vi "Query Limit Test Status.vi"(8 "error in (no error)":errorcluster, 9 "Limit Number (1: Limit 1)":i32(ring)=1 items=["Limit 1"=1, "Limit 2"=2], 10 "Function (0: Voltage DC)":i32(ring) items=["Voltage DC", "Voltage AC", "Current DC", "Current AC", "Resistance", "4-wire Resistance", "Diode", "Capacitance", "Temperature", "Continuity", "Frequency", "Period", "Voltage Ratio", "Digitize Voltage", "Digitize Current"], 11 "VISA resource name":refnum<visa-resource-name>) -> (0 "error out":errorcluster, 1 "Pass":bool, 2 "Fail Reason":string, 3 "VISA resource name out":refnum<visa-resource-name>)   [LabVIEW 2023, in "Keithley DMM6500 DAQ6500 Series.lvlib"]
doc: "Queries if the test result for limit Y should be cleared automatically or not."
uses:
  <instrlib>/Keithley DMM6500 DAQ6500 Series/Keithley DMM6500 DAQ6500 Series.lvlib
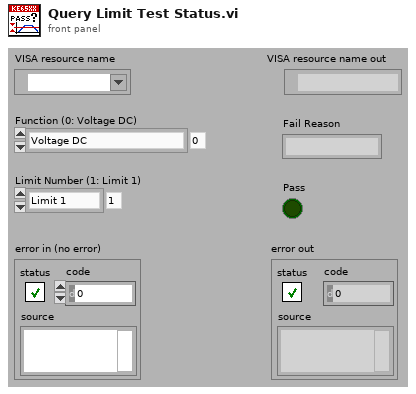
[diagram p1: front panel]
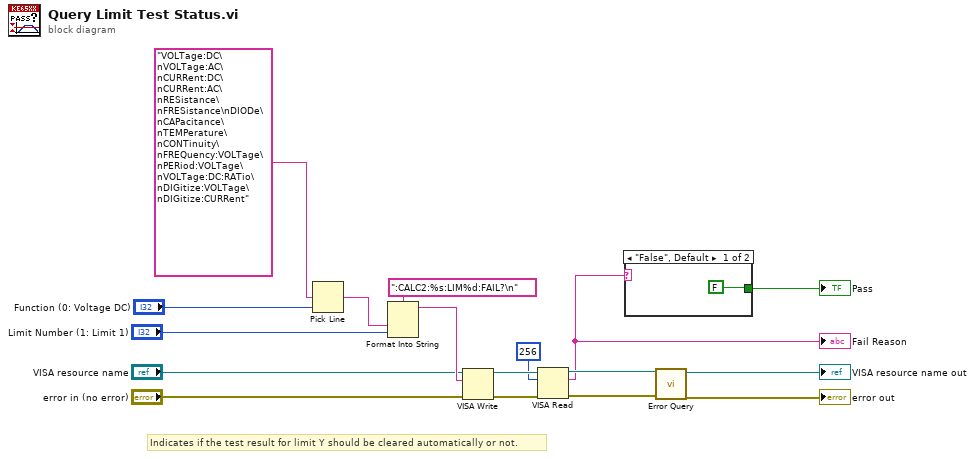
[diagram p0: block diagram]
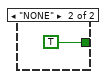
[diagram p2: hidden frame]
diagram:
  # "Indicates if the test result for limit Y should be cleared automatically or not."
  n1 = Pick Line(multi-line string="VOLTage:DC\nVOLTage:AC\nCURRent:DC\nCURRent:AC\nRESistance\nFRESistance\nDIODe\nCAPacitance\nTEMPerature\nCONTinuity\nFREQuency:VOLTage\nPERiod:VOLTage\nVOLTage:DC:RATio\nDIGitize:VOLTage\nDIGitize:CURRent", line index="Function (0: Voltage DC)") -> (output string=w9:string)  [unwired: 1 in]
  n2 = Format Into String(format string=":CALC2:%s:LIM%d:FAIL?\n", w9, "Limit Number (1: Limit 1)") -> (resulting string=w16:string)  [unwired: 2 in, 1 out]
  n3 = VISA Write(VISA resource name="VISA resource name", write buffer=w16, error in (no error)="error in (no error)") -> (VISA resource name out=w8:refnum<visa-resource-name>, error out=w6:errorcluster)  [unwired: 1 out]
  n4 = VISA Read(VISA resource name=w8, byte count=u32 256, error in (no error)=w6) -> (VISA resource name out=w7:refnum<visa-resource-name>, read buffer=w3:string, error out=w5:errorcluster)  [unwired: 1 out]
  "Fail Reason" <- w3
  n5 = case shown="\"False\", Default" w3 {
    tunnel: [FALSE ("Pass") TRUE ("Pass")] -> w2
    frame "False", Default {
    }
    frame "NONE" {
    }
  }
  "Pass" <- w2
  n6 = call <instrlib>:"Error Query.vi"("error in (no error)"=w5, "VISA resource name"=w7) -> ("error out"=→"error out":errorcluster, "VISA resource name out"=→"VISA resource name out":refnum<visa-resource-name>)  [unwired: 6 in, 2 out]
